vi "epx_Vector_Grids.vi"(9 "Plot Area Size":cluster{"Width":u32, "Height":u32}={"Width"=300, "Height"=300}, 10 "Number of Circle Grids":i32=4 min=1 max=100 step=1, 11 "Number of Polar Grids":i32=12 min=1 max=100 step=1) -> (3 "Grids":cluster{dbl[], dbl[]})   [LabVIEW 2011, in "NI_EP_Basic.lvlib" / "EPX Vector Diagram.xctl"]
uses:
  <vilib>/addons/Electrical Power/Basic/Controls/Vector Diagram/EPX Vector Diagram.xctl
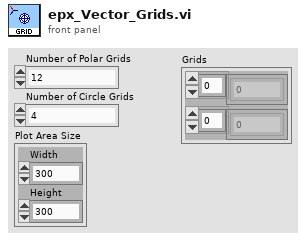
[diagram p1: front panel]
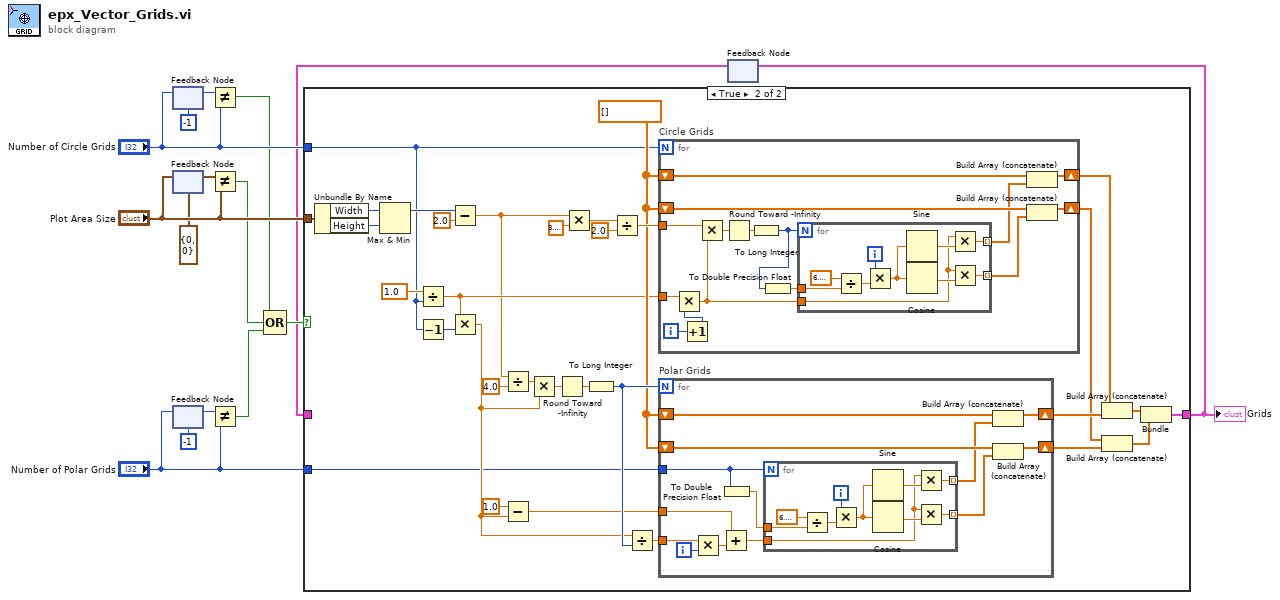
[diagram p0: block diagram]
diagram:
  n1 = feedback-in #1("Number of Circle Grids") -> ()
  n2 = feedback #1(-1 ("Number of Circle Grids")) -> (w14:i32)
  n3 = feedback-in #2("Plot Area Size") -> ()
  n4 = feedback #2(cluster{"Width":u32, "Height":u32} {"Width"=0, "Height"=0} ("Plot Area Size")) -> (w9:cluster{"Width":u32, "Height":u32})
  n5 = feedback-in #3("Number of Polar Grids") -> ()
  n6 = feedback #3(-1 ("Number of Circle Grids")) -> (w12:i32)
  n7 = Not Equal?(x=w14, y="Number of Circle Grids") -> (x != y?=w6:bool)
  n8 = Not Equal?(x=w9, y="Plot Area Size") -> (x != y?=w5:bool)
  n9 = Not Equal?(x=w12, y="Number of Polar Grids") -> (x != y?=w4:bool)
  n10 = Compound Arithmetic op=OR(w6, w5, w4) -> (w3:bool)
  n11 = feedback #4() -> (w1:cluster{dbl[], dbl[]})  [unwired: 1 in]
  n12 = case shown="True" w3 {
    tunnel: [w16 w46] -> w2
    tunnel: "Number of Circle Grids" -> [_ w19]
    tunnel: "Number of Polar Grids" -> [_ w18]
    tunnel: "Plot Area Size" -> [_ w17]
    tunnel: w1 -> [w16 _]
    frame False {
    }
    frame True {
      w32 = dbl[] []
      n13 = Unbundle By Name(w17) -> ("Width"=w22:u32, "Height"=w21:u32)
      n14 = Max & Min(x=w22, y=w21) -> (max(x,y)=w20:u32)  [unwired: 1 out]
      n15 = Divide(x=1.0, y=w19) -> (x/y=w31:dbl)
      n16 = Decrement(x=w19) -> (x-1=w33:i32)
      n17 = Subtract(x=w20, y=2.0) -> (x-y=w23:dbl)
      n18 = Multiply(x=w31, y=w33) -> (x*y=w27:dbl)
      n19 = Divide(x=w23, y=4.0) -> (x/y=w29:dbl)
      n20 = Subtract(x=1.0, y=w27) -> (x-y=w25:dbl)
      n21 = Multiply(x=w29, y=w27) -> (x*y=w28:dbl)
      n22 = Round Toward -Infinity(1:w28) -> (0:w39:dbl)
      n23 = Multiply(x=w23, y=3.141592653589793) -> (x*y=w43:dbl)
      n24 = To Long Integer(number=w39) -> (32bit integer=w38:i32)
      n25 = Divide(x=w43, y=2.0) -> (x/y=w41:dbl)
      n26 = Divide(x=w27, y=w38) -> (x/y=w40:dbl)
      n27 = for "Circle Grids" {
        N: w19 -> [_]
        shift-right: [w82] -> w37
        shift-left: w32 -> [w86]
        shift-right: [w81] -> w35
        shift-left: w32 -> [w85]
        tunnel: w31 -> [w80]
        tunnel: w41 -> [w77]
        i -> [w79]
        n28 = Increment(x=w79) -> (x+1=w72:i32)
        n29 = Multiply(x=w80, y=w72) -> (x*y=w78:dbl)
        n30 = Multiply(x=w77, y=w78) -> (x*y=w75:dbl)
        n31 = Round Toward -Infinity(1:w75) -> (0:w76:dbl)
        n32 = To Long Integer(number=w76) -> (32bit integer=w74:i32)
        n33 = To Double Precision Float(number=w74) -> (double precision float=w73:dbl)
        n34 = for {
          N: w74 -> [_]
          tunnel: [w94] -> w83 mode=indexing
          tunnel: [w93] -> w84 mode=indexing
          tunnel: w78 -> [w92]
          tunnel: w73 -> [w87]
          i -> [w89]
          n35 = Divide(x=6.283185307179586, y=w87) -> (x/y=w88:dbl)
          n36 = Multiply(x=w89, y=w88) -> (x*y=w91:dbl)
          n37 = Sine(x=w91) -> (sin(x)=w96:dbl)
          n38 = Cosine(x=w91) -> (cos(x)=w95:dbl)
          n39 = Multiply(x=w92, y=w96) -> (x*y=w94:dbl)
          n40 = Multiply(x=w92, y=w95) -> (x*y=w93:dbl)
        }
        n41 = Build Array (concatenate)(w86, w83) -> (w82:dbl[])
        n42 = Build Array (concatenate)(w85, w84) -> (w81:dbl[])
      }
      n43 = for "Polar Grids" {
        N: w38 -> [_]
        shift-right: [w57] -> w36
        shift-left: w32 -> [w61]
        shift-right: [w56] -> w34
        shift-left: w32 -> [w60]
        tunnel: w40 -> [w53]
        tunnel: w18 -> [w55]
        tunnel: w25 -> [w52]
        i -> [w50]
        n44 = Multiply(x=w53, y=w50) -> (x*y=w49:dbl)
        n45 = Add(x=w52, y=w49) -> (x+y=w51:dbl)
        n46 = To Double Precision Float(number=w55) -> (double precision float=w54:dbl)
        n47 = for {
          N: w55 -> [_]
          tunnel: [w69] -> w58 mode=indexing
          tunnel: [w68] -> w59 mode=indexing
          tunnel: w51 -> [w67]
          tunnel: w54 -> [w62]
          i -> [w64]
          n48 = Divide(x=6.283185307179586, y=w62) -> (x/y=w63:dbl)
          n49 = Multiply(x=w64, y=w63) -> (x*y=w66:dbl)
          n50 = Sine(x=w66) -> (sin(x)=w71:dbl)
          n51 = Cosine(x=w66) -> (cos(x)=w70:dbl)
          n52 = Multiply(x=w67, y=w71) -> (x*y=w69:dbl)
          n53 = Multiply(x=w67, y=w70) -> (x*y=w68:dbl)
        }
        n54 = Build Array (concatenate)(w61, w58) -> (w57:dbl[])
        n55 = Build Array (concatenate)(w60, w59) -> (w56:dbl[])
      }
      n56 = Build Array (concatenate)(w37, w36) -> (w47:dbl[])
      n57 = Build Array (concatenate)(w35, w34) -> (w48:dbl[])
      n58 = Bundle(w47, w48) -> (w46:cluster{dbl[], dbl[]})  [unwired: 1 in]
    }
  }
  "Grids" <- w2
  n59 = feedback-in #4(w2) -> ()
